vi "Read Saving.vi"(8 "error in (no error)":errorcluster, 11 "Update Caller with File State in":refnum<class "Update Caller with File State.lvclass">) -> (0 "error out":errorcluster, 2 "Saving":bool, 3 "Update Caller with File State out":refnum<class "Update Caller with File State.lvclass">)   [LabVIEW 2014, in "File Library.lvlib" / "Update Caller with File State.lvclass"]
uses:
  Update Caller with File State.lvclass
  Update Caller with File State.lvclass/Update Caller with File State.ctl
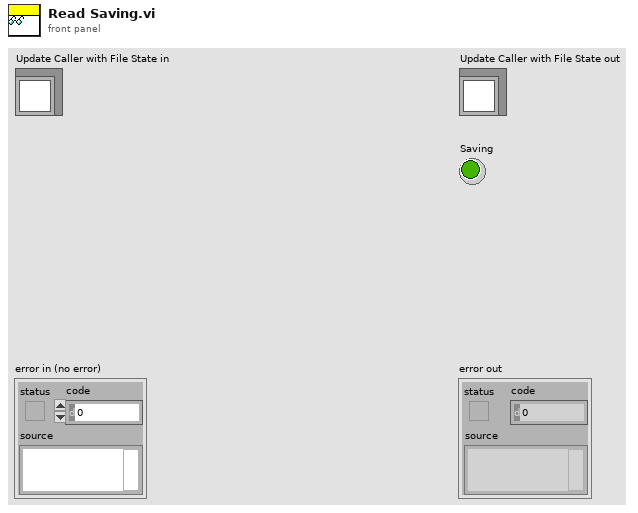
[diagram p1: front panel]
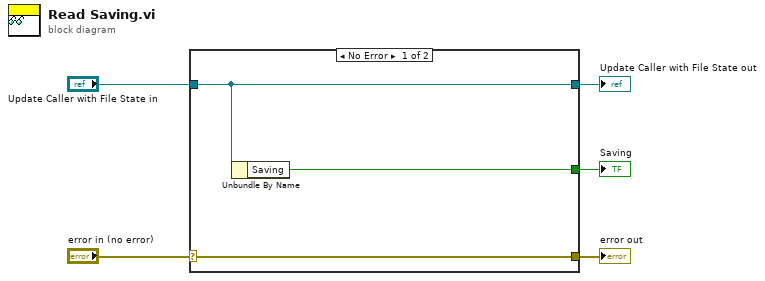
[diagram p0: block diagram]
diagram:
  n1 = case shown="No Error" "error in (no error)" {
    selector: "error in (no error)" -> [w8 w9]
    tunnel: [w8 w9] -> w4
    tunnel: [w7 w10] -> w2
    tunnel: "Update Caller with File State in" -> [w7 w10]
    tunnel: [w6 _] -> w1
    frame No Error {
      n2 = Unbundle By Name(w7) -> ("Saving"=w6:bool)
    }
    frame Error {
    }
  }
  "error out" <- w4
  "Update Caller with File State out" <- w2
  "Saving" <- w1
